vi "gather_calibration_data.vi"(6 "mode":bool, 10 "data in":T1, 11 "VISA Refnum in":refnum<visa-resource-name>) -> (1 "next timeout (ms)":i32, 2 "data out":T1, 3 "VISA Refnum out":refnum<visa-resource-name>)   [LabVIEW 2019, in "Nano33BLE-TiltCompensationSupport.lvlib"]
uses:
  types/calibrate_data.ctl
  types/xyz_array.ctl
  types/xyz.ctl
  Nano33BLE-TiltCompensationSupport.lvlib
  <vilib>/ptbypt/NI_PtbyPt.lvlib
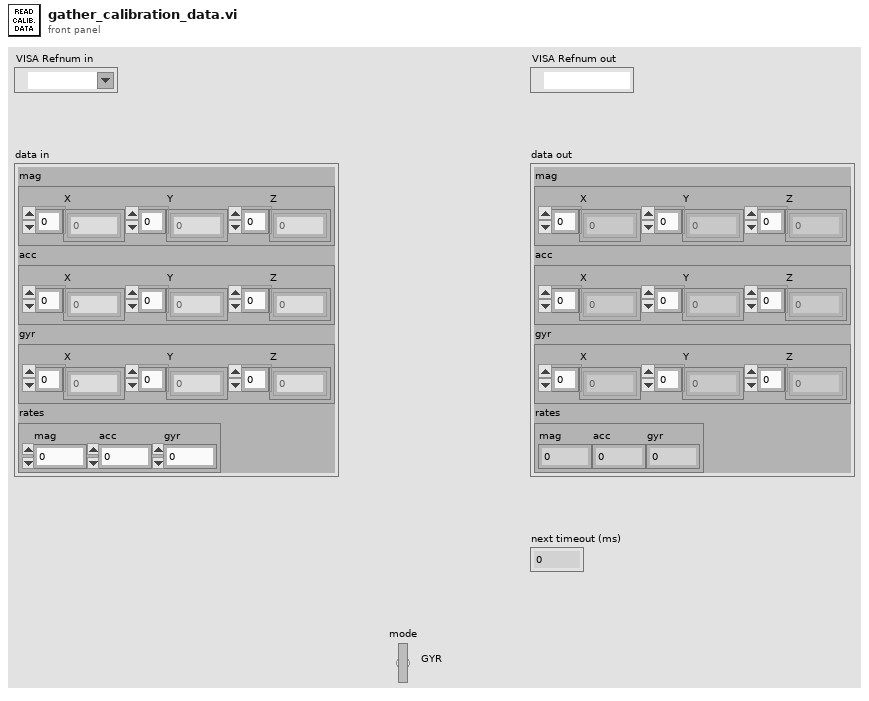
[diagram p1: front panel]
types:
  T1 = typedef "Nano33BLE-TiltCompensationSupport.lvlib/calibrate_data.ctl" = cluster{"mag":T2, "acc":T2, "gyr":T2, "rates":cluster{"mag":dbl, "acc":dbl, "gyr":dbl}}
  T2 = typedef "Nano33BLE-TiltCompensationSupport.lvlib/xyz_array.ctl" = cluster{"X":dbl[], "Y":dbl[], "Z":dbl[]}
  T3 = typedef "Nano33BLE-TiltCompensationSupport.lvlib/xyz.ctl" = cluster{"x":dbl, "y":dbl, "z":dbl}
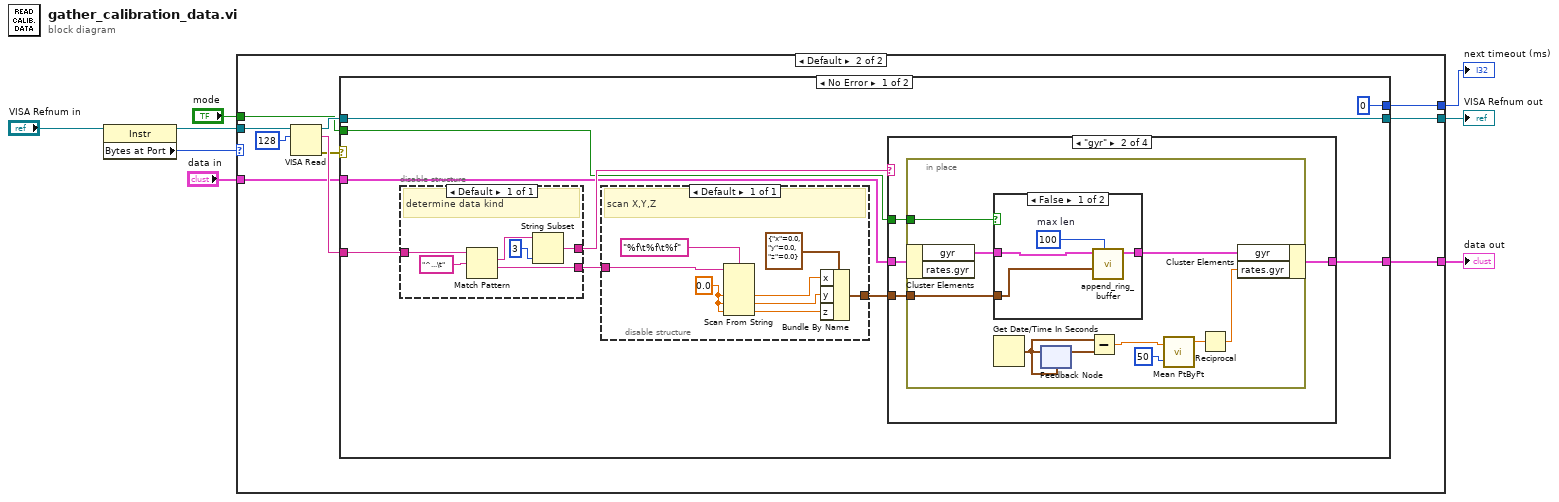
[diagram p0: block diagram]
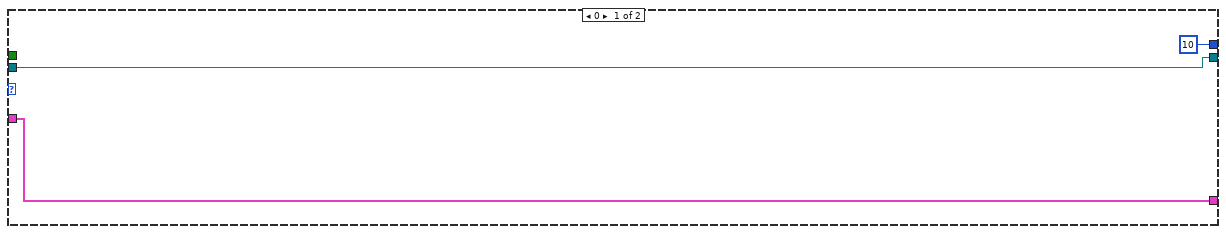
[diagram p2: hidden frame]
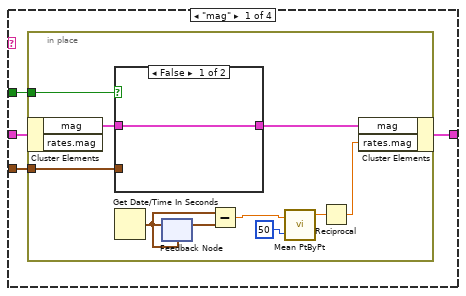
[diagram p3: hidden frame]
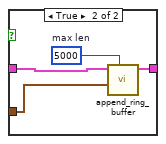
[diagram p4: hidden frame]
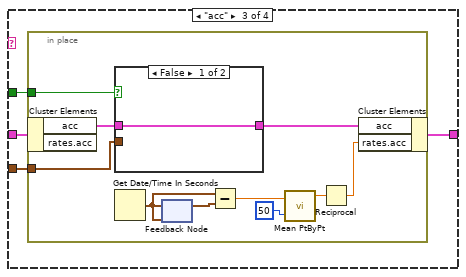
[diagram p6: hidden frame]
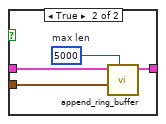
[diagram p7: hidden frame]
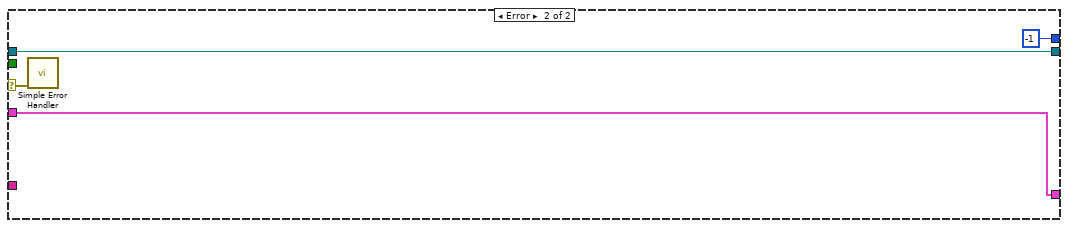
[diagram p9: hidden frame]
diagram:
  n1 = property class="Instr"(reference="VISA Refnum in") -> (reference out=w4:refnum<visa-resource-name>, "Bytes at Port"=w3:u32)  [unwired: 1 in, 1 out]
  n2 = case shown="Default" w3 {
    tunnel: w4 -> [w10 w19]
    tunnel: [10 w15] -> w5
    tunnel: [w10 w16] -> w6
    tunnel: "data in" -> [w9 w14]
    tunnel: [w9 w13] -> w8
    tunnel: "mode" -> [_ w12]
    frame 0 {
    }
    frame Default {
      n3 = VISA Read(VISA resource name=w19, byte count=u32 128) -> (VISA resource name out=w17:refnum<visa-resource-name>, read buffer=w20:string, error out=w18:errorcluster)  [unwired: 1 in, 1 out]
      n4 = case shown="No Error" w18 {
        selector: w18 -> [_ w106]
        tunnel: w20 -> [w30 _]
        tunnel: w17 -> [w28 w105]
        tunnel: [w28 w105] -> w16
        tunnel: [0 -1] -> w15
        tunnel: w14 -> [w26 w103]
        tunnel: [w25 w103] -> w13
        tunnel: w12 -> [w22 _]
        frame No Error {
          n5 = disable-structure shown="Default" {
            disable-tunnel: w30 -> [w35]
            disable-tunnel: [w32] -> w29
            disable-tunnel: [w31] -> w24
            frame Enabled {
              # "determine data kind"
              n6 = Match Pattern(string=w35, regular expression="^...\t") -> (match substring=w33:string, after substring=w31:string)  [unwired: 1 in, 2 out]
              n7 = String Subset(string=w33, length (rest)=3 ("length (rest)")) -> (substring=w32:string)  [unwired: 1 in]
            }
          }
          n8 = disable-structure shown="Default" {
            disable-tunnel: w24 -> [w42]
            disable-tunnel: [w37] -> w23
            frame Enabled {
              w43 = 0.0 ("default value 1")
              # "scan X,Y,Z"
              n9 = Scan From String(format string="%f\t%f\t%f", input string=w42, default 1=w43, default 2=w43, default 3=w43) -> (output 1=w41:dbl, output 2=w40:dbl, output 3=w39:dbl)  [unwired: 2 in, 3 out]
              n10 = Bundle By Name(cluster=T3 {"x"=0.0, "y"=0.0, "z"=0.0} ("xyz"), "x"=w41, "y"=w40, "z"=w39) -> (w37:T3)
            }
          }
          n11 = case shown="\"gyr\"" w29 {
            tunnel: w26 -> [w48 w65 w86 w102]
            tunnel: [w46 w64 w84 w102] -> w25
            tunnel: w23 -> [w47 w67 w85 _]
            tunnel: w22 -> [w45 w66 w83 _]
            frame "mag" {
              n12 = in-place {
                in-place-border: w47 -> [w57]
                in-place-border: w45 -> [w49]
                n13 = in-place-cluster #1(w48) -> ("mag"=w58:T2)  [unwired: 1 out]
                n14 = case shown="False" w49 {
                  tunnel: w58 -> [w59 w63]
                  tunnel: w57 -> [_ w62]
                  tunnel: [w59 w61] -> w56
                  frame False {
                  }
                  frame True {
                    w60 = 5000  # max len
                    n15 = call "append_ring_buffer.vi"("max len"=w60, "xyz"=w62, "data in"=w63) -> ("data out"=w61:T2)  [unwired: 8 in]
                  }
                }
                n16 = Get Date/Time In Seconds() -> (seconds since 1Jan1904=w50:timestamp)
                n17 = feedback-in #2(w50) -> ()
                n18 = feedback #2(w50) -> (w55:timestamp)
                n19 = Subtract(x=w50, y=w55) -> (x-y=w54:dbl)
                n20 = call <vilib>:"Mean PtByPt.vi"("x"=w54, "sample length"=50) -> ("mean"=w52:dbl)  [unwired: 2 in, 1 out]
                n21 = Reciprocal(x=w52) -> (1/x=w51:dbl)
                n22 = in-place-cluster #1("mag"=w56, "rates.mag"=w51) -> (w46:T1)
              }
            }
            frame "gyr" {
              n23 = in-place {
                in-place-border: w67 -> [w76]
                in-place-border: w66 -> [w68]
                n24 = in-place-cluster #3(w65) -> ("gyr"=w77:T2)  [unwired: 1 out]
                n25 = case shown="False" w68 {
                  tunnel: w77 -> [w81 w82]
                  tunnel: w76 -> [w80 _]
                  tunnel: [w79 w82] -> w75
                  frame False {
                    w78 = 100  # max len
                    n26 = call "append_ring_buffer.vi"("max len"=w78, "xyz"=w80, "data in"=w81) -> ("data out"=w79:T2)  [unwired: 8 in]
                  }
                  frame True {
                  }
                }
                n27 = Get Date/Time In Seconds() -> (seconds since 1Jan1904=w69:timestamp)
                n28 = feedback #4(w69) -> (w74:timestamp)
                n29 = feedback-in #4(w69) -> ()
                n30 = Subtract(x=w69, y=w74) -> (x-y=w73:dbl)
                n31 = call <vilib>:"Mean PtByPt.vi"("x"=w73, "sample length"=50) -> ("mean"=w72:dbl)  [unwired: 2 in, 1 out]
                n32 = Reciprocal(x=w72) -> (1/x=w70:dbl)
                n33 = in-place-cluster #3("gyr"=w75, "rates.gyr"=w70) -> (w64:T1)
              }
            }
            frame "acc" {
              n34 = in-place {
                in-place-border: w85 -> [w95]
                in-place-border: w83 -> [w87]
                n35 = in-place-cluster #5(w86) -> ("acc"=w96:T2)  [unwired: 1 out]
                n36 = case shown="False" w87 {
                  tunnel: w96 -> [w97 w101]
                  tunnel: w95 -> [_ w100]
                  tunnel: [w97 w99] -> w94
                  frame False {
                  }
                  frame True {
                    w98 = 5000  # max len
                    n37 = call "append_ring_buffer.vi"("max len"=w98, "xyz"=w100, "data in"=w101) -> ("data out"=w99:T2)  [unwired: 8 in]
                  }
                }
                n38 = Get Date/Time In Seconds() -> (seconds since 1Jan1904=w88:timestamp)
                n39 = feedback #6(w88) -> (w93:timestamp)
                n40 = feedback-in #6(w88) -> ()
                n41 = Subtract(x=w88, y=w93) -> (x-y=w92:dbl)
                n42 = call <vilib>:"Mean PtByPt.vi"("x"=w92, "sample length"=50) -> ("mean"=w91:dbl)  [unwired: 2 in, 1 out]
                n43 = Reciprocal(x=w91) -> (1/x=w89:dbl)
                n44 = in-place-cluster #5("acc"=w94, "rates.acc"=w89) -> (w84:T1)
              }
            }
            frame Default {
            }
          }
        }
        frame Error {
          n45 = call <vilib>:"Simple Error Handler.vi"("error in (no error)"=w106) -> ()  [unwired: 4 in, 5 out]
        }
      }
    }
  }
  "data out" <- w8
  "VISA Refnum out" <- w6
  "next timeout (ms)" <- w5
